vi "Get Class Child Count.vi"(8 "error in (no error)":errorcluster, 11 "Base Class Name":string) -> (0 "error out":errorcluster, 1 "Success?":bool, 2 "Class has Children?":bool, 3 "Child Count":i32)   [LabVIEW 2020, in "ClassLoader.lvlib"]
doc: "Return the number of children for the given class.\n\nThis VI does not automatically load data. Front-load before calling this VI!"
uses:
  ClassLoader.lvlib
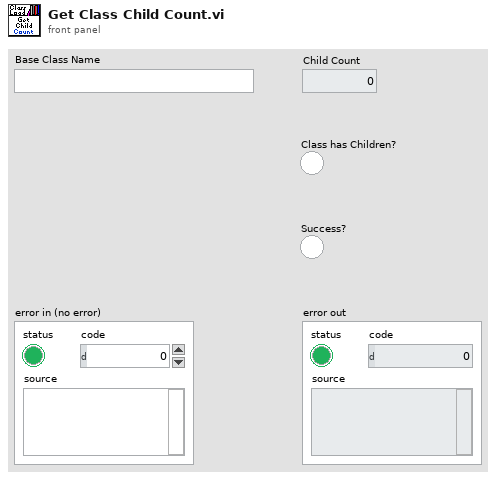
[diagram p1: front panel]
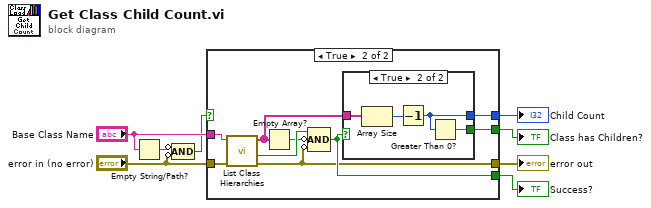
[diagram p0: block diagram]
diagram:
  n1 = Empty String/Path?(string/path="Base Class Name") -> (empty?=w3:bool)
  n2 = Compound Arithmetic op=AND(invert w3, invert "error in (no error)") -> (w4:bool)
  n3 = case shown="True" w4 {
    tunnel: "Base Class Name" -> [_ w18]
    tunnel: [w9 w10] -> w8
    tunnel: [_ w11] -> w7
    tunnel: [_ w13] -> w6
    tunnel: [_ w14] -> w2
    tunnel: "error in (no error)" -> [w9 w12]
    frame False {
    }
    frame True {
      n4 = call "List Class Hierarchies.vi"("error in (no error)"=w12, "Hierarchy Filter(empty=all)"=w18) -> ("error out"=w10:errorcluster, "Success?"=w16:bool, "Classes found"=w17:string[])  [unwired: 6 in, 1 out]
      n5 = Empty Array?(array=w17) -> (empty?=w15:bool)
      n6 = Compound Arithmetic op=AND(w16, invert w15, invert w10) -> (w11:bool)
      n7 = case shown="True" w11 {
        tunnel: w17 -> [_ w21]
        tunnel: [_ w20] -> w14
        tunnel: [_ w19] -> w13
        frame False {
        }
        frame True {
          n8 = Array Size(array=w21) -> (size(s)=w22:i32)
          n9 = Decrement(x=w22) -> (x-1=w20:i32)
          n10 = Greater Than 0?(x=w20) -> (x > 0?=w19:bool)
        }
      }
    }
  }
  "error out" <- w8
  "Success?" <- w7
  "Class has Children?" <- w6
  "Child Count" <- w2
